vi "Trigger Controls - copy saved in case Shaun screwed up a revised version.vi"() -> ()   [LabVIEW 2012]
panel:
  out "Final Output":T1
  in  "Set Point Alt":dbl=8000.0 min=0.0 max=10000.0 step=1.0
  out "Force Output":T1
  out "Numeric Control":i32=1
  in  "Stop Button":bool
  in  "Tab Control":enum32{"CO2", "AD"}(tab)=enum."AD"
  in  "High CO2 Forces":T1={"Main 1"=TRUE, "Main 2"=TRUE, "Recirc  3"=FALSE, "Boost A 7"=TRUE, "Recirc  9"=FALSE, "Scrub 4"=TRUE, "Scrub 10"=TRUE, "O2 5"=FALSE, "Vent 6"=TRUE, "Boost A 8"=TRUE, "Vent 11"=TRUE, "Boost B 12"=TRUE, "Boost B 13"=TRUE, "Recirc 14"=FALSE, "Scrub 15"=TRUE, "Vent 16"=TRUE, "Main 17"=TRUE, "Boost A 18"=TRUE, "Boost B 19"=TRUE, "Boost F 20"=TRUE, "Vent 2 21"=TRUE}
  in  "Run C1":T2={"Main 1"=inf, "Main 2"=inf, "Recirc  3"=9000.0, "Boost A 7"=3400.0, "Recirc  9"=9000.0, "Scrub 4"=8800.0, "Scrub 10"=8800.0, "O2 5"=9600.0, "Vent 6"=9200.0, "Boost A 8"=3400.0, "Vent 11"=9200.0, "Boost B 12"=1800.0, "Boost B 13"=1800.0, "Recirc 14"=9000.0, "Scrub 15"=8800.0, "Vent 16"=9200.0, "Main 17"=inf, "Boost A 18"=3400.0, "Boost B 19"=1800.0, "Boost F 20"=7000.0, "Vent 2 21"=9200.0}
  in  "Run C2":T2={"Main 1"=inf, "Main 2"=inf, "Recirc  3"=8800.0, "Boost A 7"=3000.0, "Recirc  9"=8800.0, "Scrub 4"=8600.0, "Scrub 10"=8600.0, "O2 5"=9600.0, "Vent 6"=9000.0, "Boost A 8"=3000.0, "Vent 11"=9000.0, "Boost B 12"=1400.0, "Boost B 13"=1400.0, "Recirc 14"=8800.0, "Scrub 15"=8600.0, "Vent 16"=9000.0, "Main 17"=inf, "Boost A 18"=3000.0, "Boost B 19"=1400.0, "Boost F 20"=6600.0, "Vent 2 21"=9000.0}
  in  "Hold C3":T2={"Main 1"=1800.0, "Main 2"=1800.0, "Recirc  3"=9000.0, "Boost A 7"=3400.0, "Recirc  9"=9000.0, "Scrub 4"=8800.0, "Scrub 10"=8800.0, "O2 5"=9600.0, "Vent 6"=9200.0, "Boost A 8"=3400.0, "Vent 11"=9200.0, "Boost B 12"=1800.0, "Boost B 13"=1800.0, "Recirc 14"=9000.0, "Scrub 15"=8800.0, "Vent 16"=9200.0, "Main 17"=1800.0, "Boost A 18"=3400.0, "Boost B 19"=1800.0, "Boost F 20"=7000.0, "Vent 2 21"=9200.0}
  in  "Hold C4":T2={"Main 1"=1400.0, "Main 2"=1400.0, "Recirc  3"=8800.0, "Boost A 7"=3000.0, "Recirc  9"=8800.0, "Scrub 4"=8600.0, "Scrub 10"=8600.0, "O2 5"=9600.0, "Vent 6"=9000.0, "Boost A 8"=3000.0, "Vent 11"=9000.0, "Boost B 12"=1400.0, "Boost B 13"=1400.0, "Recirc 14"=8800.0, "Scrub 15"=8600.0, "Vent 16"=9000.0, "Main 17"=1400.0, "Boost A 18"=3000.0, "Boost B 19"=1400.0, "Boost F 20"=6600.0, "Vent 2 21"=9000.0}
  out "Force State":T1
  in  "CO2 ppm":dbl(slide) scale=0.0..10000.0 scale format="%#.0f"
  out "AD State":T1
  out "AD Output":T1
  in  "Hold A4":T2={"Main 1"=-150.0, "Main 2"=-150.0, "Recirc  3"=-30.0, "Boost A 7"=-250.0, "Recirc  9"=-30.0, "Scrub 4"=inf, "Scrub 10"=inf, "O2 5"=80.0, "Vent 6"=15.0, "Boost A 8"=-250.0, "Vent 11"=15.0, "Boost B 12"=-300.0, "Boost B 13"=-300.0, "Recirc 14"=-30.0, "Scrub 15"=inf, "Vent 16"=15.0, "Main 17"=-150.0, "Boost A 18"=-250.0, "Boost B 19"=-300.0, "Boost F 20"=-300.0, "Vent 2 21"=650.0}
  in  "Hold A3":T2={"Main 1"=0.0, "Main 2"=0.0, "Recirc  3"=50.0, "Boost A 7"=-150.0, "Recirc  9"=50.0, "Scrub 4"=inf, "Scrub 10"=inf, "O2 5"=150.0, "Vent 6"=60.0, "Boost A 8"=-150.0, "Vent 11"=60.0, "Boost B 12"=-200.0, "Boost B 13"=-200.0, "Recirc 14"=50.0, "Scrub 15"=inf, "Vent 16"=60.0, "Main 17"=0.0, "Boost A 18"=-150.0, "Boost B 19"=-200.0, "Boost F 20"=-200.0, "Vent 2 21"=700.0}
  in  "Run A1":T2={"Main 1"=inf, "Main 2"=inf, "Recirc  3"=-30.0, "Boost A 7"=-80.0, "Recirc  9"=-30.0, "Scrub 4"=inf, "Scrub 10"=inf, "O2 5"=80.0, "Vent 6"=15.0, "Boost A 8"=-80.0, "Vent 11"=15.0, "Boost B 12"=-50.0, "Boost B 13"=-50.0, "Recirc 14"=-30.0, "Scrub 15"=inf, "Vent 16"=15.0, "Main 17"=inf, "Boost A 18"=0.0, "Boost B 19"=-50.0, "Boost F 20"=-80.0, "Vent 2 21"=650.0}
  in  "High AD Diff":T1={"Main 1"=FALSE, "Main 2"=FALSE, "Recirc  3"=FALSE, "Boost A 7"=FALSE, "Recirc  9"=FALSE, "Scrub 4"=TRUE, "Scrub 10"=TRUE, "O2 5"=FALSE, "Vent 6"=TRUE, "Boost A 8"=FALSE, "Vent 11"=TRUE, "Boost B 12"=FALSE, "Boost B 13"=FALSE, "Recirc 14"=FALSE, "Scrub 15"=TRUE, "Vent 16"=TRUE, "Main 17"=FALSE, "Boost A 18"=FALSE, "Boost B 19"=FALSE, "Boost F 20"=FALSE, "Vent 2 21"=TRUE}
  in  "Delay S":T2={"Main 1"=30.0, "Main 2"=30.0, "Recirc  3"=1.0, "Boost A 7"=30.0, "Recirc  9"=1.0, "Scrub 4"=1.0, "Scrub 10"=1.0, "O2 5"=1.0, "Vent 6"=1.0, "Boost A 8"=30.0, "Vent 11"=1.0, "Boost B 12"=30.0, "Boost B 13"=30.0, "Recirc 14"=1.0, "Scrub 15"=1.0, "Vent 16"=1.0, "Main 17"=30.0, "Boost A 18"=30.0, "Boost B 19"=30.0, "Boost F 20"=30.0, "Vent 2 21"=1.0}
  in  "Run A1":T2={"Main 1"=inf, "Main 2"=inf, "Recirc  3"=50.0, "Boost A 7"=0.0, "Recirc  9"=50.0, "Scrub 4"=inf, "Scrub 10"=inf, "O2 5"=150.0, "Vent 6"=60.0, "Boost A 8"=0.0, "Vent 11"=60.0, "Boost B 12"=15.0, "Boost B 13"=15.0, "Recirc 14"=50.0, "Scrub 15"=inf, "Vent 16"=60.0, "Main 17"=inf, "Boost A 18"=0.0, "Boost B 19"=15.0, "Boost F 20"=0.0, "Vent 2 21"=700.0}
  in  "Alt Dif M":dbl(slide)=1000.0 scale=-1000.0..1000.0
  in  "Set Point Force":T2={"Main 1"=inf, "Main 2"=inf, "Recirc  3"=inf, "Boost A 7"=inf, "Recirc  9"=inf, "Scrub 4"=inf, "Scrub 10"=inf, "O2 5"=inf, "Vent 6"=inf, "Boost A 8"=inf, "Vent 11"=inf, "Boost B 12"=inf, "Boost B 13"=inf, "Recirc 14"=inf, "Scrub 15"=inf, "Vent 16"=inf, "Main 17"=inf, "Boost A 18"=inf, "Boost B 19"=inf, "Boost F 20"=6000.0, "Vent 2 21"=inf}
  in  "Mode":enum16{"Run", "Hold", "Off"}(ring)=enum."Off"
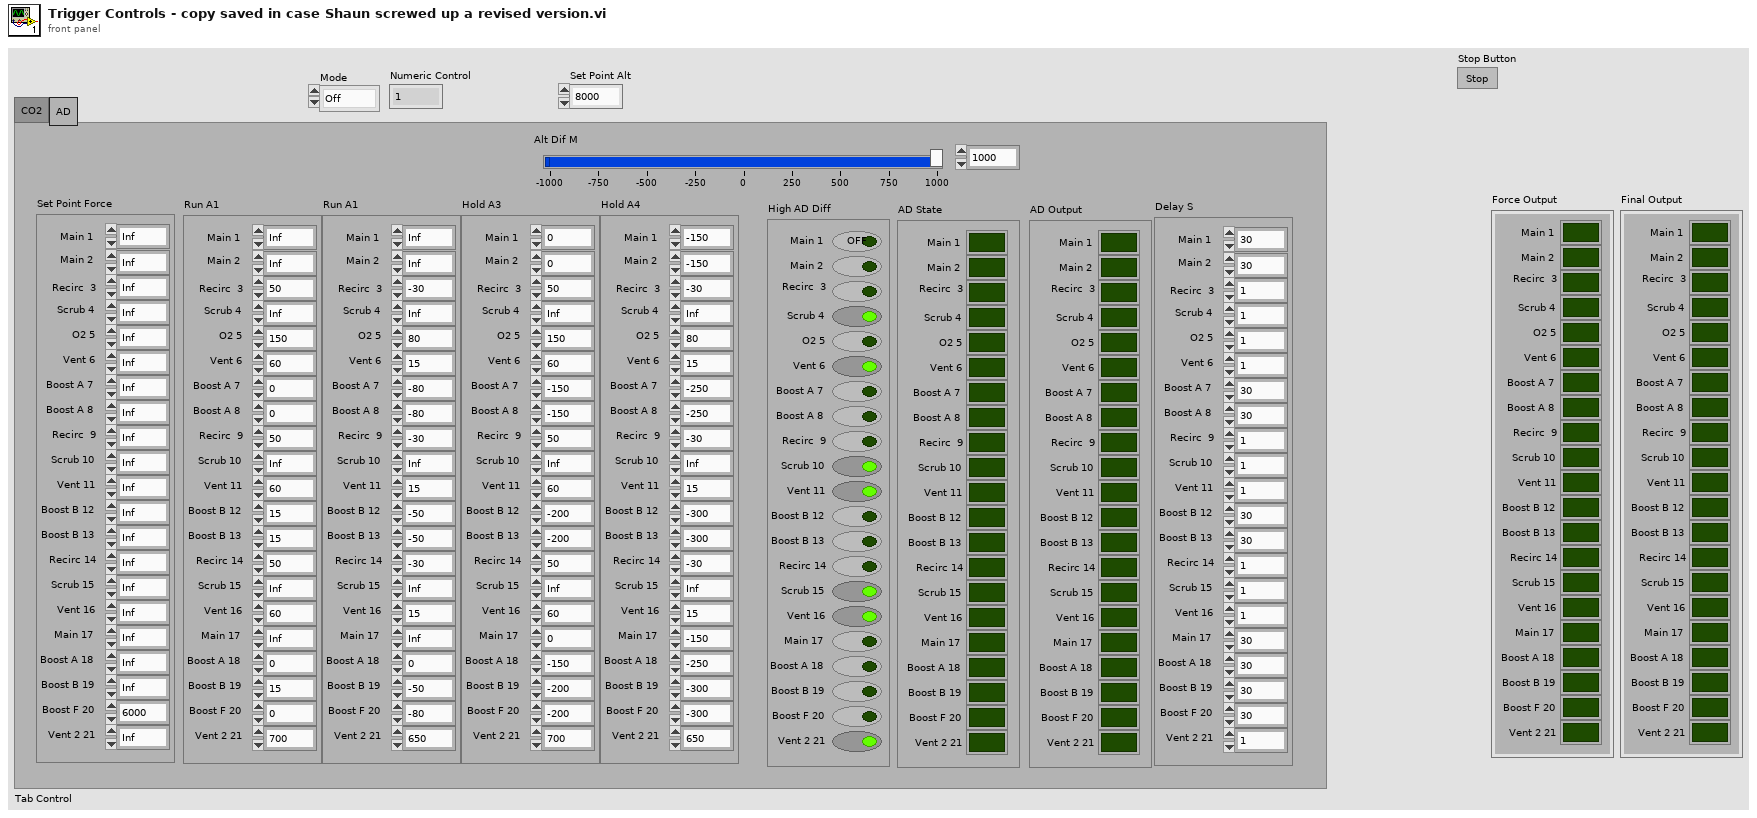
[diagram p1: front panel]
types:
  T1 = cluster{"Main 1":bool, "Main 2":bool, "Recirc  3":bool, "Boost A 7":bool, "Recirc  9":bool, "Scrub 4":bool, "Scrub 10":bool, "O2 5":bool, "Vent 6":bool, "Boost A 8":bool, "Vent 11":bool, "Boost B 12":bool, "Boost B 13":bool, "Recirc 14":bool, "Scrub 15":bool, "Vent 16":bool, "Main 17":bool, "Boost A 18":bool, "Boost B 19":bool, "Boost F 20":bool, "Vent 2 21":bool}
  T2 = cluster{"Main 1":dbl, "Main 2":dbl, "Recirc  3":dbl, "Boost A 7":dbl, "Recirc  9":dbl, "Scrub 4":dbl, "Scrub 10":dbl, "O2 5":dbl, "Vent 6":dbl, "Boost A 8":dbl, "Vent 11":dbl, "Boost B 12":dbl, "Boost B 13":dbl, "Recirc 14":dbl, "Scrub 15":dbl, "Vent 16":dbl, "Main 17":dbl, "Boost A 18":dbl, "Boost B 19":dbl, "Boost F 20":dbl, "Vent 2 21":dbl}
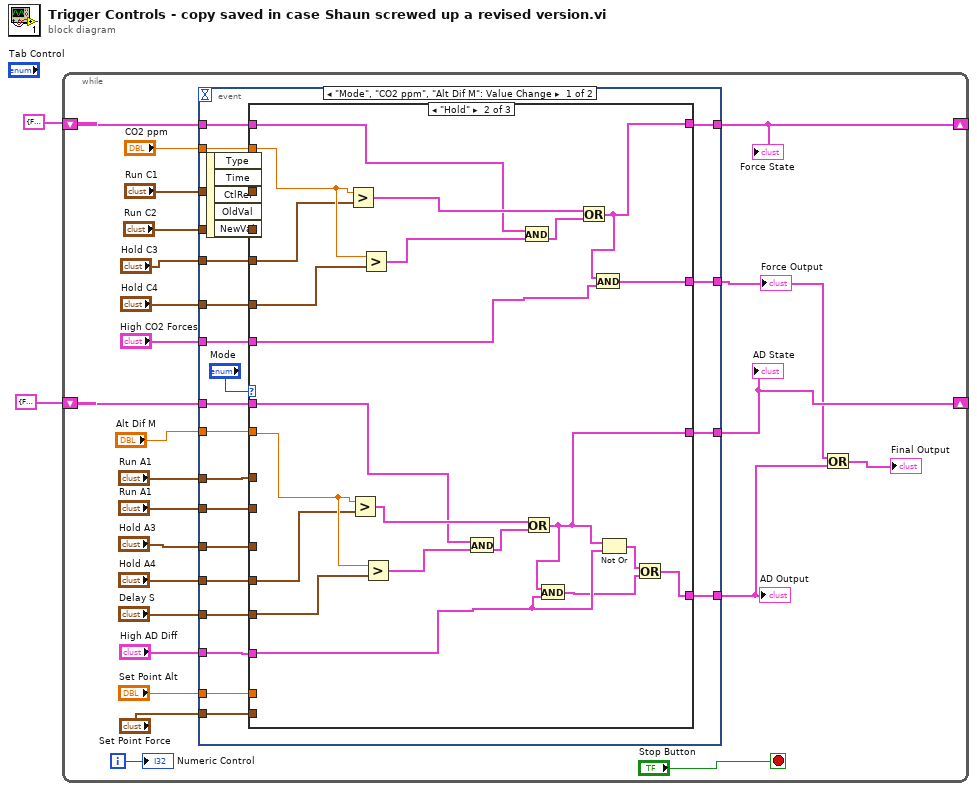
[diagram p0: block diagram]
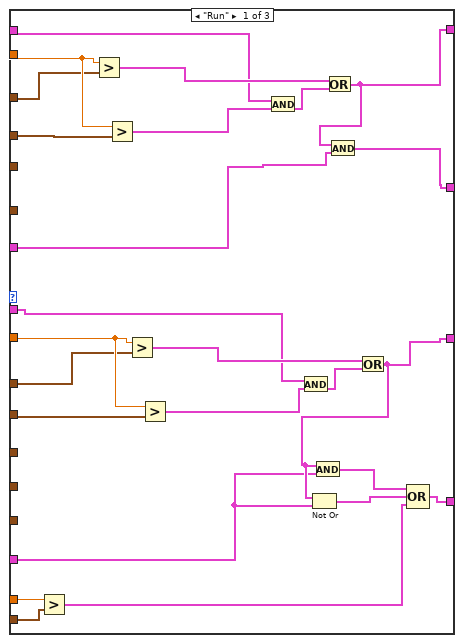
[diagram p2: hidden frame]
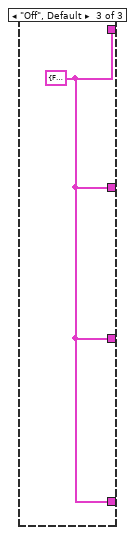
[diagram p3: hidden frame]
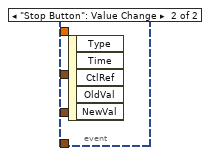
[diagram p4: hidden frame]
diagram:
  n1 = while {
    shift-right: [w21] -> _
    shift-left: T1 {"Main 1"=FALSE, "Main 2"=FALSE, "Recirc  3"=FALSE, "Boost A 7"=FALSE, "Recirc  9"=FALSE, "Scrub 4"=FALSE, "Scrub 10"=FALSE, "O2 5"=FALSE, "Vent 6"=FALSE, "Boost A 8"=FALSE, "Vent 11"=FALSE, "Boost B 12"=FALSE, "Boost B 13"=FALSE, "Recirc 14"=FALSE, "Scrub 15"=FALSE, "Vent 16"=FALSE, "Main 17"=FALSE, "Boost A 18"=FALSE, "Boost B 19"=FALSE, "Boost F 20"=FALSE, "Vent 2 21"=FALSE} -> [w19]
    shift-right: [w9] -> _
    shift-left: T1 {"Main 1"=FALSE, "Main 2"=FALSE, "Recirc  3"=FALSE, "Boost A 7"=FALSE, "Recirc  9"=FALSE, "Scrub 4"=FALSE, "Scrub 10"=FALSE, "O2 5"=FALSE, "Vent 6"=FALSE, "Boost A 8"=FALSE, "Vent 11"=FALSE, "Boost B 12"=FALSE, "Boost B 13"=FALSE, "Recirc 14"=FALSE, "Scrub 15"=FALSE, "Vent 16"=FALSE, "Main 17"=FALSE, "Boost A 18"=FALSE, "Boost B 19"=FALSE, "Boost F 20"=FALSE, "Vent 2 21"=FALSE} ("AD State") -> [w8]
    i -> [w18]
    stop <- "Stop Button" stop-if-true
    n2 = event shown="[0] \"Mode\", \"CO2 ppm\", \"Alt Dif M\": Value Change" {
      selector: _ -> [_ _]
      dyn-events: _ -> [_ _]
      timeout: _ -> [_ _]
      tunnel: "CO2 ppm" -> [w48 _]
      tunnel: "Run C1" -> [w47 _]
      tunnel: "Run C2" -> [w46 _]
      tunnel: "Hold C3" -> [w45 _]
      tunnel: "Hold C4" -> [w44 _]
      tunnel: [w43 _] -> w21
      tunnel: w19 -> [w42 _]
      tunnel: "High CO2 Forces" -> [w40 _]
      tunnel: [w39 _] -> w5
      tunnel: "Alt Dif M" -> [w38 _]
      tunnel: "Run A1" -> [w37 _]
      tunnel: "Run A1" -> [w36 _]
      tunnel: "Hold A3" -> [w35 _]
      tunnel: "Hold A4" -> [w34 _]
      tunnel: "Delay S" -> [w33 _]
      tunnel: "High AD Diff" -> [w32 _]
      tunnel: [w31 _] -> w9
      tunnel: w8 -> [w30 _]
      tunnel: [w29 _] -> w4
      tunnel: "Set Point Alt" -> [w28 _]
      tunnel: "Set Point Force" -> [w27 _]
      event "Mode", "CO2 ppm", "Alt Dif M": Value Change {
        n3 = event-data() -> ()  [unwired: 1 in, 5 out]
        n4 = case shown="\"Hold\"" "Mode" {
          tunnel: w48 -> [w72 w92 _]
          tunnel: w47 -> [w71 _ _]
          tunnel: [w61 w89 w96] -> w43
          tunnel: w46 -> [w73 _ _]
          tunnel: w45 -> [_ w91 _]
          tunnel: w44 -> [_ w90 _]
          tunnel: w42 -> [w68 w93 _]
          tunnel: w40 -> [w58 w79 _]
          tunnel: [w57 w80 w96] -> w39
          tunnel: w38 -> [w64 w86 _]
          tunnel: w37 -> [w63 _ _]
          tunnel: w36 -> [w62 _ _]
          tunnel: w35 -> [_ _ _]
          tunnel: w34 -> [_ w83 _]
          tunnel: w33 -> [_ w84 _]
          tunnel: w32 -> [w55 w77 _]
          tunnel: [w56 w78 w96] -> w31
          tunnel: w30 -> [w65 w85 _]
          tunnel: [w49 w74 w96] -> w29
          tunnel: w28 -> [w52 _ _]
          tunnel: w27 -> [w51 _ _]
          frame "Run" {
            n5 = Greater?(x=w52, y=w51) -> (0:w50:T1)
            n6 = Greater?(x=w72, y=w71) -> (0:w70:T1)
            n7 = Greater?(x=w72, y=w73) -> (0:w60:T1)
            n8 = Greater?(x=w64, y=w63) -> (0:w67:T1)
            n9 = Greater?(x=w64, y=w62) -> (0:w59:T1)
            n10 = And(x=w68, y=w60) -> (x .and. y?=w69:T1)
            n11 = And(x=w65, y=w59) -> (x .and. y?=w66:T1)
            n12 = Or(x=w70, y=w69) -> (x .or. y?=w61:T1)
            n13 = And(x=w61, y=w58) -> (x .and. y?=w57:T1)
            n14 = Or(x=w67, y=w66) -> (x .or. y?=w56:T1)
            n15 = Not Or(1:w55, 2:w56) -> (0:w53:T1)
            n16 = And(x=w56, y=w55) -> (x .and. y?=w54:T1)
            n17 = Compound Arithmetic op=OR(w54, w53, w50) -> (w49:T1)
          }
          frame "Hold" {
            n18 = Greater?(x=w92, y=w91) -> (0:w95:T1)
            n19 = Greater?(x=w86, y=w83) -> (0:w88:T1)
            n20 = Greater?(x=w92, y=w90) -> (0:w82:T1)
            n21 = Greater?(x=w86, y=w84) -> (0:w81:T1)
            n22 = And(x=w85, y=w81) -> (x .and. y?=w87:T1)
            n23 = And(x=w93, y=w82) -> (x .and. y?=w94:T1)
            n24 = Or(x=w88, y=w87) -> (x .or. y?=w78:T1)
            n25 = And(x=w78, y=w77) -> (x .and. y?=w75:T1)
            n26 = Or(x=w95, y=w94) -> (x .or. y?=w89:T1)
            n27 = And(x=w89, y=w79) -> (x .and. y?=w80:T1)
            n28 = Not Or(1:w77, 2:w78) -> (0:w76:T1)
            n29 = Or(x=w76, y=w75) -> (x .or. y?=w74:T1)
          }
          frame "Off", Default {
            w96 = T1 {"Main 1"=FALSE, "Main 2"=FALSE, "Recirc  3"=FALSE, "Boost A 7"=FALSE, "Recirc  9"=FALSE, "Scrub 4"=FALSE, "Scrub 10"=FALSE, "O2 5"=FALSE, "Vent 6"=FALSE, "Boost A 8"=FALSE, "Vent 11"=FALSE, "Boost B 12"=FALSE, "Boost B 13"=FALSE, "Recirc 14"=FALSE, "Scrub 15"=FALSE, "Vent 16"=FALSE, "Main 17"=FALSE, "Boost A 18"=FALSE, "Boost B 19"=FALSE, "Boost F 20"=FALSE, "Vent 2 21"=FALSE}
          }
        }
      }
      event "Stop Button": Value Change {
        n30 = event-data() -> ()  [unwired: 1 in, 5 out]
      }
    }
    "Force State" <- w21
    "Force Output" <- w5
    "AD State" <- w9
    "AD Output" <- w4
    n31 = Or(x=w5, y=w4) -> (x .or. y?=→"Final Output":T1)
    "Numeric Control" <- w18
  }
